vi "Request Data.vi"(8 "error in":errorcluster) -> (0 "error out":errorcluster, 3 "Response Queue":refnum<queue>)   [LabVIEW 2019, in "ASCII Actor.lvlib"]
uses:
  ASCII Actor.lvlib
  Actor Task.ctl
  Actor Command.ctl
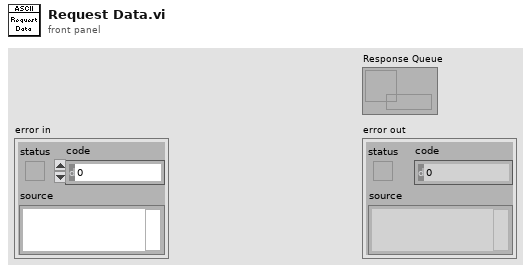
[diagram p1: front panel]
types:
  T1 = typedef "ASCII Actor.lvlib/Actor Task.ctl" = enum8{"Write", "Get Data", "Stop"}
  T2 = typedef "ASCII Actor.lvlib/Actor Command.ctl" = cluster{"Task":T1, "Data":string, "Response Queue":refnum<queue>}
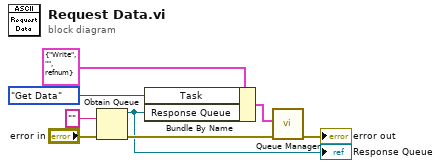
[diagram p0: block diagram]
diagram:
  n1 = Obtain Queue(element data type="", error in (no error)="error in") -> (queue out=w1:refnum<queue>, error out=w6:errorcluster)  [unwired: 3 in, 1 out]
  "Response Queue" <- w1
  n2 = Bundle By Name(cluster=T2 {"Task"=enum."Write", "Data"="", "Response Queue"=refnum} ("Command"), "Task"=Actor_Task."Get Data", "Response Queue"=w1) -> (w3:T2)
  n3 = call "Queue Manager.vi"("error in"=w6, "Command"=w3) -> ("error out"=→"error out":errorcluster)  [unwired: 8 in, 1 out]
